vi "Test Disable Plugins.vi"(8 "error in (no error)":errorcluster, 11 "Configuration Manager Test in":refnum<class "Configuration Manager Test.lvclass">) -> (0 "error out":errorcluster, 3 "Configuration Manager Test out":refnum<class "Configuration Manager Test.lvclass">)   [LabVIEW 2020, in "Configuration Manager Test.lvclass"]
uses:
  Configuration Manager Test.lvclass
  Configuration Manager Test.lvclass/Configuration Manager Test.ctl
  source/User Interface/Configuration Manager/Configuration Manager.lvclass
  b78b68b9-28ec-4fcb-9b61-f705c7f0904e.vi
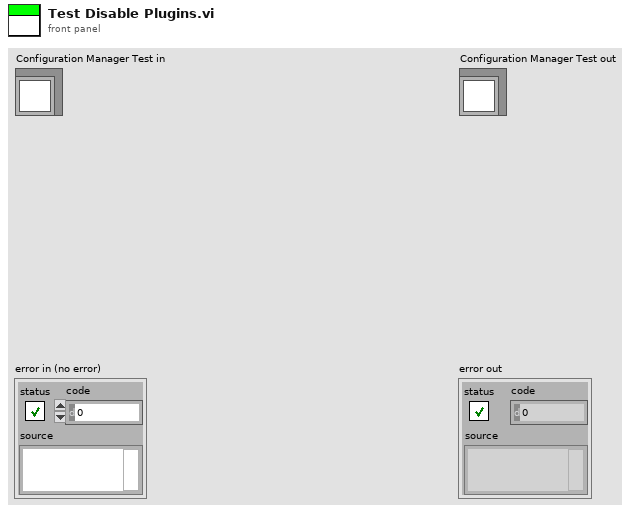
[diagram p1: front panel]
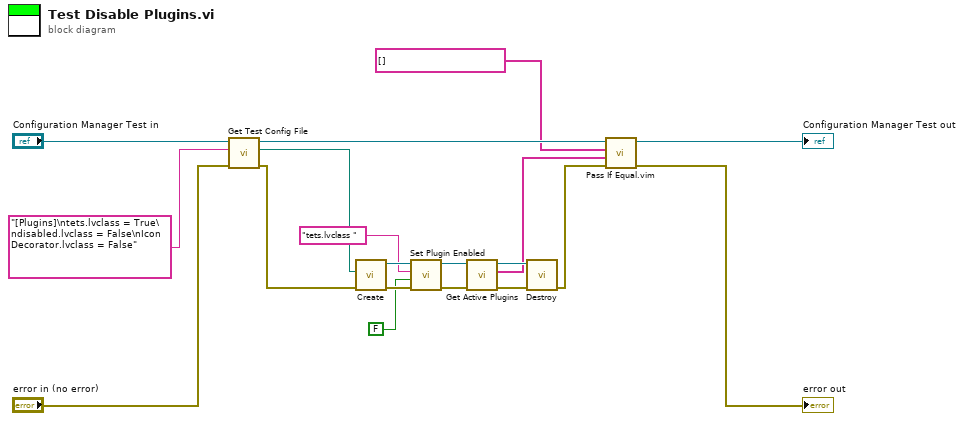
[diagram p0: block diagram]
diagram:
  n1 = call "Get Test Config File.vi"("error in (no error)"="error in (no error)", "File Content"="[Plugins]\ntets.lvclass = True\ndisabled.lvclass = False\nIcon Decorator.lvclass = False", "Configuration Manager Test in"="Configuration Manager Test in") -> ("error out"=w13:errorcluster, "File Path"=w9:path, "Configuration Manager Test out"=w2:refnum<class "Configuration Manager Test.lvclass">)  [unwired: 6 in]
  n2 = call "Create.vi"("error in (no error)"=w13, "configuration file path"=w9) -> ("error out"=w16:errorcluster, "Configuration Manager out"=w6:refnum<class "Configuration Manager.lvclass">)  [unwired: 8 in]
  n3 = call "Set Plugin Enabled.vi"("error in (no error)"=w16, "Enabled?"=FALSE, "Plugin"="tets.lvclass ", "Configuration Manager in"=w6) -> ("error out"=w7:errorcluster, "Configuration Manager out"=w5:refnum<class "Configuration Manager.lvclass">)  [unwired: 6 in]
  n4 = call "Get Active Plugins.vi"("error in (no error)"=w7, "Configuration Manager In"=w5) -> ("error out"=w14:errorcluster, "Plugins"=w8:string[], "Configuration Manager Out"=w15:refnum<class "Configuration Manager.lvclass">)  [unwired: 7 in]
  n5 = call "Destroy.vi"("error in (no error)"=w14, "Configuration Manager In"=w15) -> ("error out"=w12:errorcluster)  [unwired: 9 in]
  n6 = call "Pass If Equal.vim"("error in (no error)"=w12, "Actual"=w8, "Expected"=string[] [], "LUnit Test Case In"=w2) -> ("error out"=→"error out":errorcluster, "LUnit Test Case Out"=→"Configuration Manager Test out":refnum<class "Configuration Manager Test.lvclass">)  [unwired: 6 in]
